vi "Set_NMeas.vi"(0 "VisaCluster":T1, 7 "measured values":i32, 11 "error in (no error)":errorcluster) -> (4 "VisaCluster":T1, 8 "measure values":string, 15 "error out":errorcluster)   [LabVIEW 2014, in "FH 55.lvlib"]
doc: "This VI sets how many measure values must be displayed and gives the measure values out."
uses:
  FH 55.lvlib
  TypeDef/VisaCluster.ctl
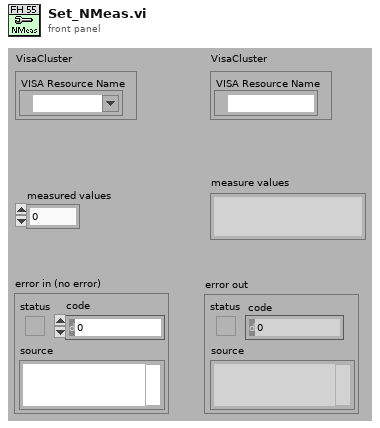
[diagram p1: front panel]
types:
  T1 = typedef "FH 55.lvlib/VisaCluster.ctl" = cluster{"VISA Resource Name":refnum<visa-resource-name>}
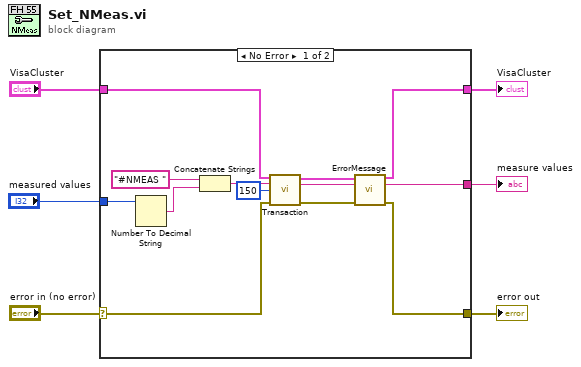
[diagram p0: block diagram]
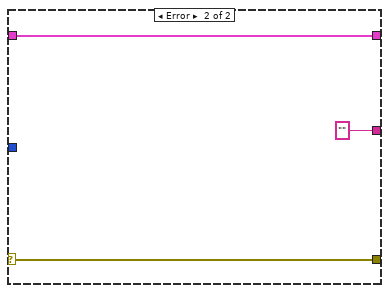
[diagram p2: hidden frame]
diagram:
  n1 = case shown="No Error" "error in (no error)" {
    selector: "error in (no error)" -> [w15 w21]
    tunnel: "VisaCluster" -> [w16 w22]
    tunnel: "measured values" -> [w11 _]
    tunnel: [w19 w22] -> w2
    tunnel: [w17 w21] -> w4
    tunnel: [w18 ""] -> w3
    frame No Error {
      n2 = Number To Decimal String(number=w11) -> (decimal integer string=w10:string)  [unwired: 1 in]
      n3 = Concatenate Strings("#NMEAS " ("string"), w10) -> (w8:string)
      n4 = call "Transaction.vi"("VisaCluster"=w16, "Command"=w8, "Time (150) ms"=u32 150, "error in (no error)"=w15) -> ("VisaCluster"=w12:T1, "Answer"=w13:string, "error out"=w14:errorcluster)  [unwired: 8 in, 1 out]
      n5 = call "ErrorMessage.vi"("VisaCluster"=w12, "Message In"=w13, "error in (no error)"=w14) -> ("VisaCluster"=w19:T1, "Message Out"=w18:string, "error out"=w17:errorcluster)  [unwired: 10 in]
    }
    frame Error {
    }
  }
  "error out" <- w4
  "measure values" <- w3
  "VisaCluster" <- w2
